vi "Generate_random_password.vi"(8 "error in (no error)":errorcluster caption="错误输入（无错误）") -> (0 "error out":errorcluster caption="错误输出", 3 "Generate random password":string)   [LabVIEW 2016]
panel:
  out "无符号字节数组":u8[](array[numeric])
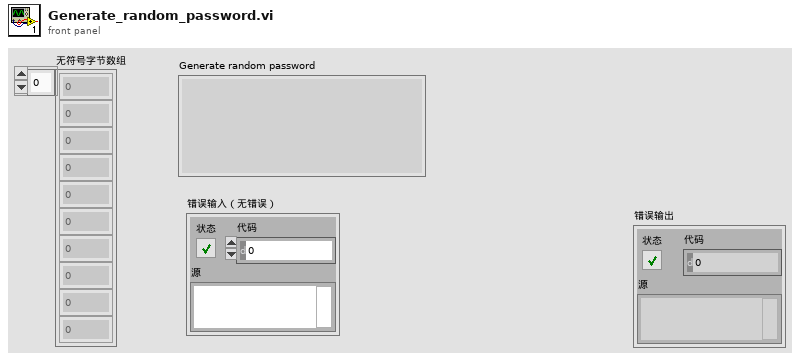
[diagram p1: front panel]
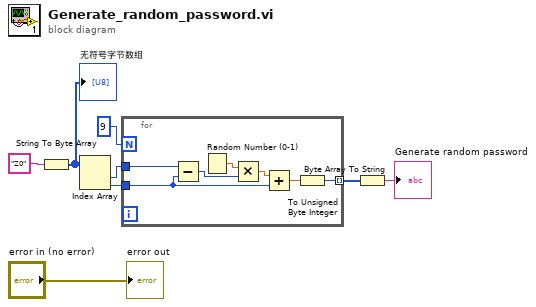
[diagram p0: block diagram]
diagram:
  n1 = String To Byte Array(string="Z0" ("字符串")) -> (unsigned byte array=w6:u8[])
  "无符号字节数组" <- w6
  n2 = Index Array(array=w6) -> (element #1=w5:u8, element #2=w4:u8)  [unwired: 2 in]
  n3 = for {
    N: 9 -> [_]
    tunnel: w5 -> [w14]
    tunnel: w4 -> [w11]
    tunnel: [w9] -> w3 mode=indexing
    n4 = Subtract(x=w14, y=w11) -> (x-y=w13:u8)
    n5 = Random Number (0-1)() -> (number: 0 to 1=w15:dbl)
    n6 = Multiply(x=w15, y=w13) -> (x*y=w12:dbl)
    n7 = Add(x=w12, y=w11) -> (x+y=w10:dbl)
    n8 = To Unsigned Byte Integer(number=w10) -> (unsigned 8bit integer=w9:u8)
  }
  n9 = Byte Array To String(unsigned byte array=w3) -> (string=→"Generate random password":string)
  "error out" <- "error in (no error)"
